vi "Launcher.vi"   [LabVIEW 2020]
uses:
  Supervisor/Supervisor/Supervisor.lvclass
  <vilib>/ActorFramework/Actor/Actor.lvclass
types:
  T1 = enum32{"Invalid", "Standard", "Closed", "Hidden", "Minimized", "Maximized"}
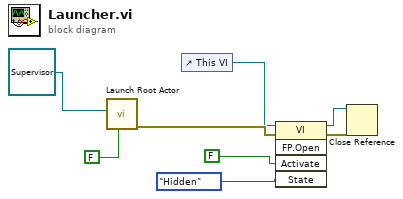
[diagram p0: block diagram]
diagram:
  n1 = call <vilib>:"Launch Root Actor.vi"("Open Actor Core front panel? (F)"=FALSE, "Actor"=refnum<class "Supervisor.lvclass"> refnum ("Supervisor.lvlib:Supervisor.lvclass")) -> ("error out"=w6:errorcluster)  [unwired: 8 in, 1 out]
  n2 = control-ref of="This VI"() -> (w5:refnum<vi>)
  n3 = invoke class="VI" method="FP.Open"(reference=w5, error in=w6, "Activate"=FALSE ("Activate?"), "State"=T1."Hidden") -> (reference out=w1:refnum<vi>, error out=w2:errorcluster)  [unwired: 1 in, 3 out]
  n4 = Close Reference(reference=w1, error in (no error)=w2) -> ()  [unwired: 1 out]
